vi "Read Data - DTL (Scalar).vi"(5 "Data Block #":u16, 8 "error in (no error)":errorcluster, 9 "Start Address":T1, 10 "Memory Area":T2 items=["P Area"=128, "I Area"=129, "O Area"=130, "M Area"=131, "DB Area"=132, "Counter"=40, "Timer"=41], 11 "S7 in":refnum<class "S7NetCom.lvclass">) -> (0 "error out":errorcluster, 2 "Time Stamp":timestamp, 3 "S7 out":refnum<class "S7NetCom.lvclass">)   [LabVIEW 2014, in "S7NetCom.lvclass"]
doc: "Reads a single (scalar) Real value from the PLC. \n_____\nCopyright (c) 2019 Hampel Software Engineering (HSE), released under BSD license. More info can be found on https://dokuwiki.hampel-soft.com/code/hse/s7netcom. Original code published by Marc Christenson, Sisu Devices."
uses:
  S7NetCom.lvclass
  Controls/S7_Variable_Type.ctl
  Controls/S7_Memory_Area.ctl
  Controls/S7_Start_Address.ctl
panel:
  # "More info on https://dokuwiki.hampel-soft.com/code/hse/s7netcom\n\nCopyright (c) 2019, HAMPEL SOFTWARE ENGINEERING (HSE)\nOriginal code developed by Marc Christenson, Sisu Devices\nAll rights reserved.\n\nRedistribution and use in source and binary forms, with or without\nmodification, are permitted provided that the following conditions are met:\n\n1. Redistributions of source code must retain the above copyright\n   notice, this list of conditions and the following disclaimer.\n\n2. Redistributions in binary form must reproduce the above copyright\n   notice, this list of conditions and the following disclaimer in the\n   documentation and/or other materials provided with the distribution.\n\n3. All advertising materials mentioning features or use of this software\n   must display the following acknowledgement:\n   This product includes software developed by HAMPEL SOFTWARE ENGINEERING.\n\n4. Neither the name of HAMPEL SOFTWARE ENGINEERING nor the\n   names of its contributors may be used to endorse or promote products\n   derived from this software without specific prior written permission.\n\nTHIS SOFTWARE IS PROVIDED BY HAMPEL SOFTWARE ENGINEERING ''AS IS'' AND ANY\nEXPRESS OR IMPLIED WARRANTIES, INCLUDING, BUT NOT LIMITED TO, THE IMPLIED\nWARRANTIES OF MERCHANTABILITY AND FITNESS FOR A PARTICULAR PURPOSE ARE\nDISCLAIMED. IN NO EVENT SHALL HAMPEL SOFTWARE ENGINEERING BE LIABLE FOR ANY\nDIRECT, INDIRECT, INCIDENTAL, SPECIAL, EXEMPLARY, OR CONSEQUENTIAL DAMAGES\n(INCLUDING, BUT NOT LIMITED TO, PROCUREMENT OF SUBSTITUTE GOODS OR SERVICES;\nLOSS OF USE, DATA, OR PROFITS; OR BUSINESS INTERRUPTION) HOWEVER CAUSED AND\nON ANY THEORY OF LIABILITY, WHETHER IN CONTRACT, STRICT LIABILITY, OR TORT\n(INCLUDING NEGLIGENCE OR OTHERWISE) ARISING IN ANY WAY OUT OF THE USE OF THIS\nSOFTWARE, EVEN IF ADVISED OF THE POSSIBILITY OF SUCH DAMAGE."
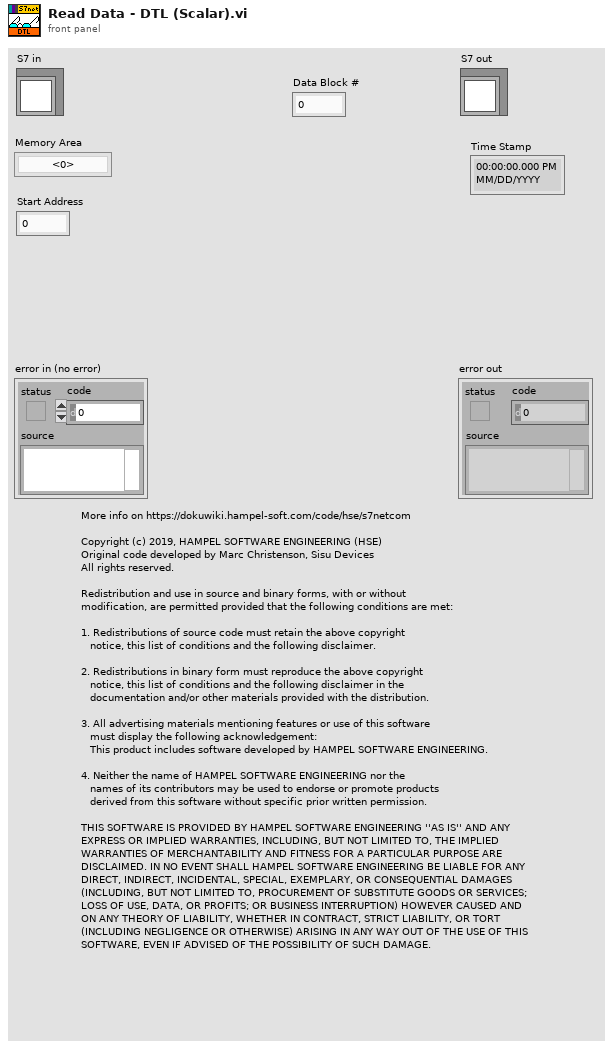
[diagram p1: front panel]
types:
  T1 = typedef "S7NetCom.lvclass/S7_Start_Address.ctl" = u16
  T2 = typedef "S7NetCom.lvclass/S7_Memory_Area.ctl" = u8
  T3 = typedef "S7NetCom.lvclass/S7_Variable_Type.ctl" = enum8{"---", "BIT", "BYTE", "CHAR", "WORD", "INT", "DWORD", "DINT", "REAL"}
  T4 = typedef "S7NetCom.lvclass/S7NetCom_HexByteArray.ctl" = T5[]
  T5 = typedef "S7NetCom.lvclass/S7NetCom_HexByte.ctl" = u8
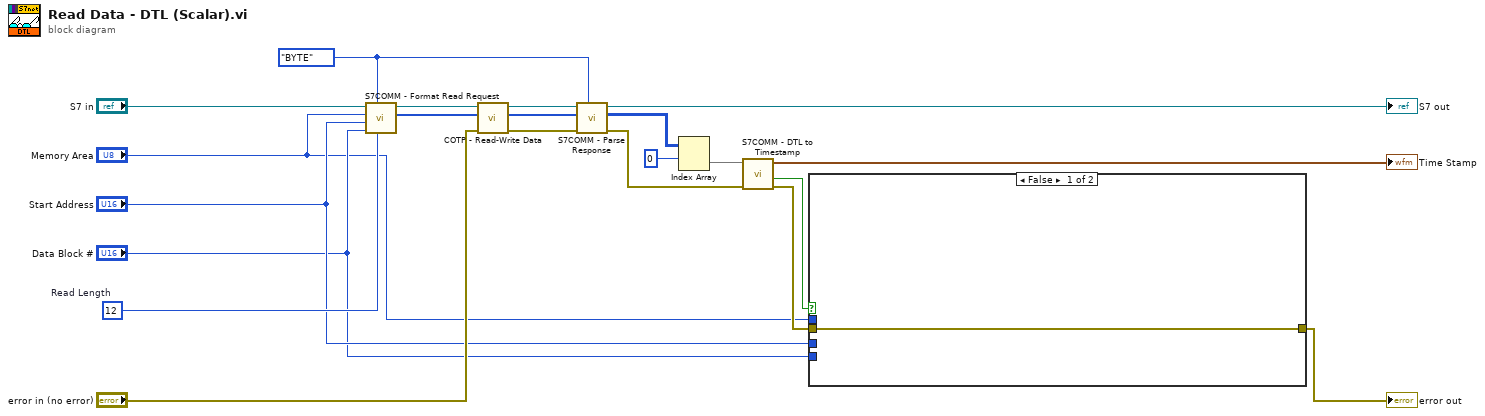
[diagram p0: block diagram]
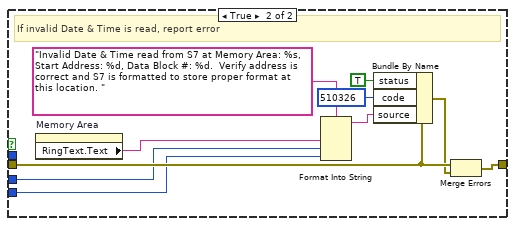
[diagram p2: hidden frame]
diagram:
  w10 = u16 12  # Read Length
  w15 = S7_Variable_Type."BYTE" ("Variable Type")
  n1 = call "S7COMM - Format Read Request.vi"("Read Length"=w10, "Variable Type"=w15, "Data Block #"="Data Block #", "Start Address"="Start Address", "Memory Area"="Memory Area", "S7"="S7 in") -> ("S7 PDU Data"=w19:T4, "S7 out"=w18:refnum<class "S7NetCom.lvclass">)  [unwired: 4 in]
  n2 = call "COTP - Read-Write Data.vi"("error in (no error)"="error in (no error)", "S7 PDU in"=w19, "S7 in"=w18) -> ("error out"=w13:errorcluster, "S7 PDU out"=w14:T4, "S7 out"=w20:refnum<class "S7NetCom.lvclass">)  [unwired: 6 in]
  n3 = call "S7COMM - Parse Response.vi"("Variable Type"=w15, "error in (no error)"=w13, "S7 PDU Data"=w14, "S7"=w20) -> ("error out"=w9:errorcluster, "Data Array"=w12:i32[][], "S7 out"=→"S7 out":refnum<class "S7NetCom.lvclass">)  [unwired: 4 in, 1 out]
  n4 = Index Array(array=w12, index (row)=0) -> (element=w8:i32[])  [unwired: 1 in]
  n5 = call "S7COMM - DTL to Timestamp.vi"("error in (no error)"=w9, "S7 DTL"=w8) -> ("error out"=w5:errorcluster, "Invalid Timestamp"=w6:bool, "Time Stamp"=→"Time Stamp":timestamp)  [unwired: 6 in, 1 out]
  n6 = case shown="False" w6 {
    tunnel: w5 -> [w22 w31]
    tunnel: [w22 w32] -> w4
    tunnel: "Data Block #" -> [_ w26]
    tunnel: "Start Address" -> [_ w27]
    tunnel: "Memory Area" -> [_ _]
    frame False {
    }
    frame True {
      # "If invalid Date & Time is read, report error"
      n7 = property on="Memory Area" class="Ring (strict)"() -> ("RingText.Text"=w28:string)  [unwired: 2 in, 2 out]
      n8 = Format Into String(format string="Invalid Date & Time read from S7 at Memory Area: %s, Start Address: %d, Data Block #: %d.  Verify address is correct and S7 is formatted to store proper format at this location. ", w28, w27, w26) -> (resulting string=w24:string)  [unwired: 2 in, 1 out]
      n9 = Bundle By Name(cluster=w31, "status"=TRUE, "code"=510326, "source"=w24) -> (w23:errorcluster)
      n10 = Merge Errors(w31, w23) -> (w32:errorcluster)
    }
  }
  "error out" <- w4
